vi "Send TX Message.vi"(8 "error in (no error)":errorcluster, 11 "RxTx in":refnum<class "RxTx.lvclass">) -> (0 "error out":errorcluster, 3 "RxTx out":refnum<class "RxTx.lvclass">)   [LabVIEW 2018, in "RxTx.lvclass"]
doc: "Send Tx message"
uses:
  RxTx.lvclass
  RxTx.lvclass/RxTx.ctl
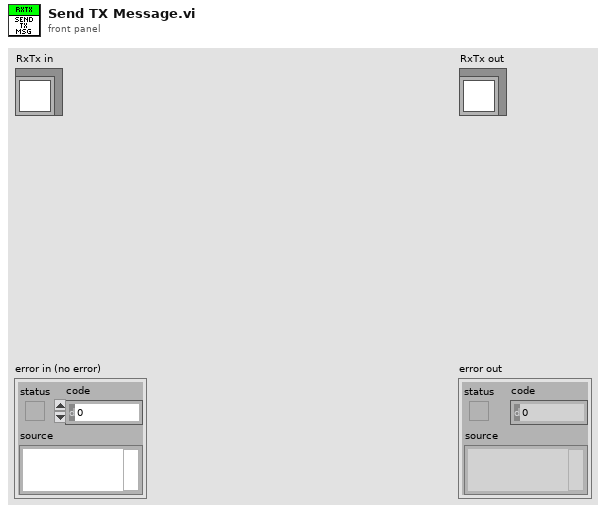
[diagram p1: front panel]
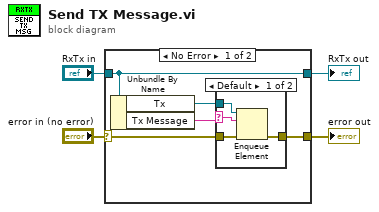
[diagram p0: block diagram]
diagram:
  n1 = case shown="No Error" "error in (no error)" {
    selector: "error in (no error)" -> [w8 w16]
    tunnel: [w6 w16] -> w3
    tunnel: [w7 w15] -> w1
    tunnel: "RxTx in" -> [w7 w15]
    frame No Error {
      n2 = Unbundle By Name(w7) -> ("Tx"=w9:refnum<queue>, "Tx Message"=w5:string)
      n3 = case shown="Default" w5 {
        selector: w5 -> [w10 _]
        tunnel: w9 -> [w13 _]
        tunnel: w8 -> [w12 w14]
        tunnel: [w11 w14] -> w6
        frame Default {
          n4 = Enqueue Element(queue=w13, element=w10, error in (no error)=w12) -> (error out=w11:errorcluster)  [unwired: 1 in, 2 out]
        }
        frame "" {
        }
      }
    }
    frame Error {
    }
  }
  "error out" <- w3
  "RxTx out" <- w1
